vi "Set Current Protection.vi"(8 "error in":errorcluster, 11 "3300 in":refnum<class "3300.lvclass">) -> (0 "error out":errorcluster, 3 "3300 out":refnum<class "3300.lvclass">)   [LabVIEW 2019, in "3300.lvlib" / "3300.lvclass"]
uses:
  Library/3300.lvclass
  C:/Users/Public/Documents/Development/builds/Instruments/Electronic Load.lvlibp/Library/Electronic Load.lvclass
  Library/3300.lvclass/3300.ctl
  Accessors/Read Local Resource.vi
  Accessors/Write Local Resource.vi
  builds/Instruments/Electronic Load.lvlibp/Accessors/Protection/Read OCP Enable.vi
  builds/Instruments/Electronic Load.lvlibp/Accessors/Protection/Read OCP Level.vi
  builds/Instruments/Electronic Load.lvlibp/Accessors/Protection/Read OCP Delay.vi
  <instrlib>/Agilent N330X Series/Agilent N330X Series.lvlib
  builds/Engine/Engine.lvlibp/Project/Engine.lvclass
  C:/Users/Public/Documents/Development/builds/Engine/Engine.lvlibp/Project/Engine.lvclass
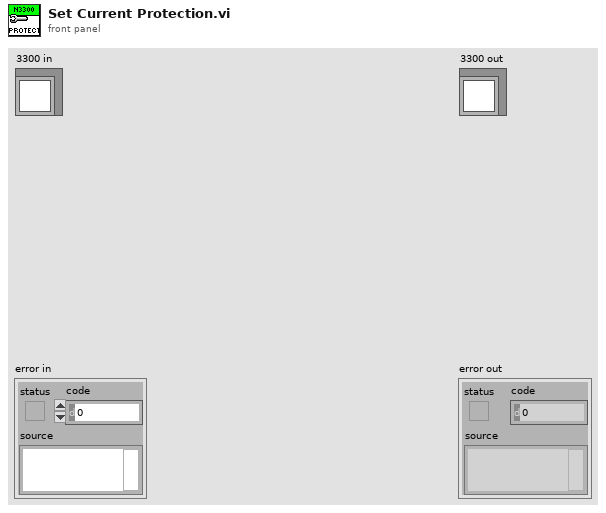
[diagram p1: front panel]
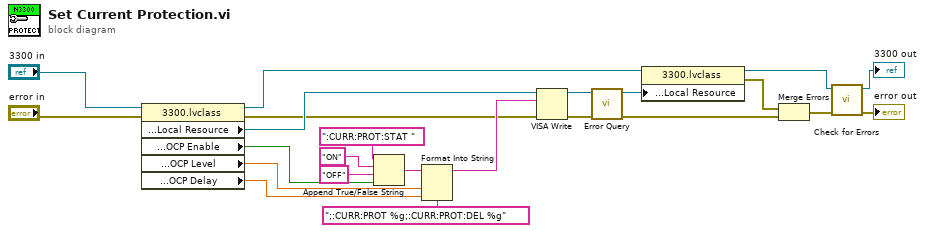
[diagram p0: block diagram]
diagram:
  n1 = property class="3300.lvclass"(reference="3300 in", error in="error in") -> (reference out=w20:refnum<class "3300.lvclass">, error out=w6:errorcluster, "Private:Accessors:Local Resource"=w8:refnum<visa-resource-name>, "Accessors:Settings:Protection:OCP Enable"=w11:bool, "Accessors:Settings:Protection:OCP Level"=w10:dbl, "Accessors:Settings:Protection:OCP Delay"=w9:dbl)
  n2 = Append True/False String(1:w11, 2:"OFF" ("false string"), 3:"ON" ("true string"), 4:":CURR:PROT:STAT " ("format string")) -> (0:w13:string)
  n3 = Format Into String(format string=";:CURR:PROT %g;:CURR:PROT:DEL %g", initial string=w13, w10, w9) -> (resulting string=w12:string)  [unwired: 1 in, 1 out]
  n4 = VISA Write(VISA resource name=w8, write buffer=w12, error in (no error)=w6) -> (VISA resource name out=w19:refnum<visa-resource-name>, error out=w18:errorcluster)  [unwired: 1 out]
  n5 = call <instrlib>:"Error Query.vi"("error in (no error)"=w18, "VISA resource name"=w19) -> ("error out"=w5:errorcluster, "VISA resource name out"=w7:refnum<visa-resource-name>)  [unwired: 6 in, 2 out]
  n6 = property class="3300.lvclass"(reference=w20, "Private:Accessors:Local Resource"=w7) -> (reference out=w2:refnum<class "3300.lvclass">, error out=w22:errorcluster)  [unwired: 1 in]
  n7 = Merge Errors(w22, w5) -> (w4:errorcluster)
  n8 = call "Check for Errors.vi"("error in"=w4, "Engine in"=w2) -> ("error out"=→"error out":errorcluster, "Engine out"=→"3300 out":refnum<class "3300.lvclass">)  [unwired: 8 in]
